vi "Parse for Instrument Name.vi"(9 "Instrument Name":string, 10 "Message In":T1, 11 "Message Queue":refnum<queue>) -> (2 "Message Out":T1)   [LabVIEW 2013, in "Cal Inst.lvlib" / "Cal Inst Message Queue.lvlib"]
uses:
  Cal Inst Message Queue.lvlib
  Message Cluster.ctl
  <vilib>/regexp/Match Regular Expression.xnode
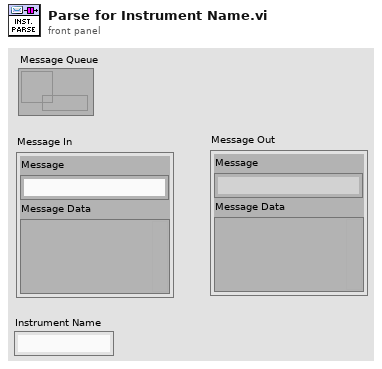
[diagram p1: front panel]
types:
  T1 = typedef "Cal Inst.lvlib/Cal Inst Message Queue.lvlib/Message Cluster.ctl" = cluster{"Message":string, "Message Data":variant}
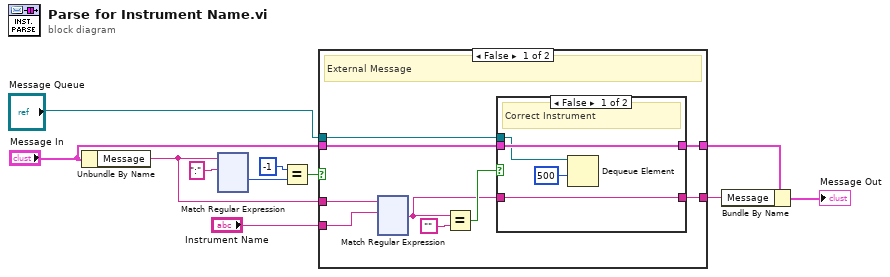
[diagram p0: block diagram]
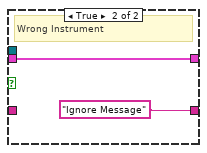
[diagram p2: hidden frame]
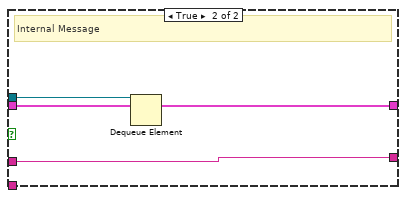
[diagram p3: hidden frame]
diagram:
  n1 = Unbundle By Name("Message In") -> ("Message"=w6:string)
  n2 = xnode "Match Regular Expression"("input string"=w6, "regular expression"=":") -> ("offset past match"=w10:i32)  [unwired: 4 in, 4 out]
  n3 = Equal?(x=-1, y=w10) -> (x = y?=w8:bool)
  n4 = case shown="False" w8 {
    tunnel: [w15 w143] -> w5
    tunnel: "Instrument Name" -> [w20 _]
    tunnel: w6 -> [w18 w143]
    tunnel: "Message Queue" -> [w14 w141]
    tunnel: "Message In" -> [w13 w142]
    tunnel: [w12 w142] -> w4
    frame False {
      # "External Message"
      n5 = xnode "Match Regular Expression"("input string"=w18, "regular expression"=w20) -> ("after match"=w16:string)  [unwired: 4 in, 4 out]
      n6 = Equal?(x=w16, y="") -> (x = y?=w17:bool)
      n7 = case shown="False" w17 {
        tunnel: w16 -> [w24 _]
        tunnel: [w24 "Ignore Message" ("t")] -> w15
        tunnel: w14 -> [w22 _]
        tunnel: w13 -> [w23 w25]
        tunnel: [w23 w25] -> w12
        frame False {
          # "Correct Instrument"
          n8 = Dequeue Element(queue=w22, timeout in ms (-1)=500) -> ()  [unwired: 1 in, 4 out]
        }
        frame True {
          # "Wrong Instrument"
        }
      }
    }
    frame True {
      # "Internal Message"
      n9 = Dequeue Element(queue=w141) -> ()  [unwired: 2 in, 4 out]
    }
  }
  n10 = Bundle By Name(cluster=w4, "Message"=w5) -> (→"Message Out":T1)
